vi "Gen - Polar Plot.vi"(4 "Lines/Points":enum16{"Lines", "Points"}(ring)=enum."Points", 5 "font":T1={"desired font(Application) "=enum."Application Font", "[user-specified font] "={"Font Name:"="", "Size"=0, "Strikeout?"=FALSE, "Italic?"=FALSE, "Underline?"=FALSE, "Outline?"=FALSE, "Shadow?"=FALSE, "Bold?"=FALSE}}, 6 "polar attributes":T2={"maximum"=0.0, "minimum"=0.0, "clip to min"=FALSE, "log?(F)"=FALSE, "grid color"=6710886, "plot color"=16711680, "fmt and prec"={"format"=enum."Decimal", "precision"=0}, "visible section"=8} {"minimum" format="%0.3f"; "maximum" format="%0.3f"}, 7 "Size":u16=1, 8 "Scale atrributes":cluster{"Scale Polar plot":dbl, "1 rev FS":dbl}={"Scale Polar plot"=0.2, "1 rev FS"=0.0} {"1 rev FS" format="%#_13g"; "Scale Polar plot" format="%#_13g"}, 9 "dimensions (w,h)":cluster{"width":i16, "height":i16}, 10 "data array [mag, phase (deg)]":cluster{"magnitude":dbl, "phase":dbl}[](array[cluster]) {"phase" format="%0.2f"; "magnitude" format="%0.2f"}, 11 "picture":picture) -> (3 "new picture":picture)   [LabVIEW 2020]
panel:
  in  "top left point(0, 0)":cluster{"x":i16, "y":i16}
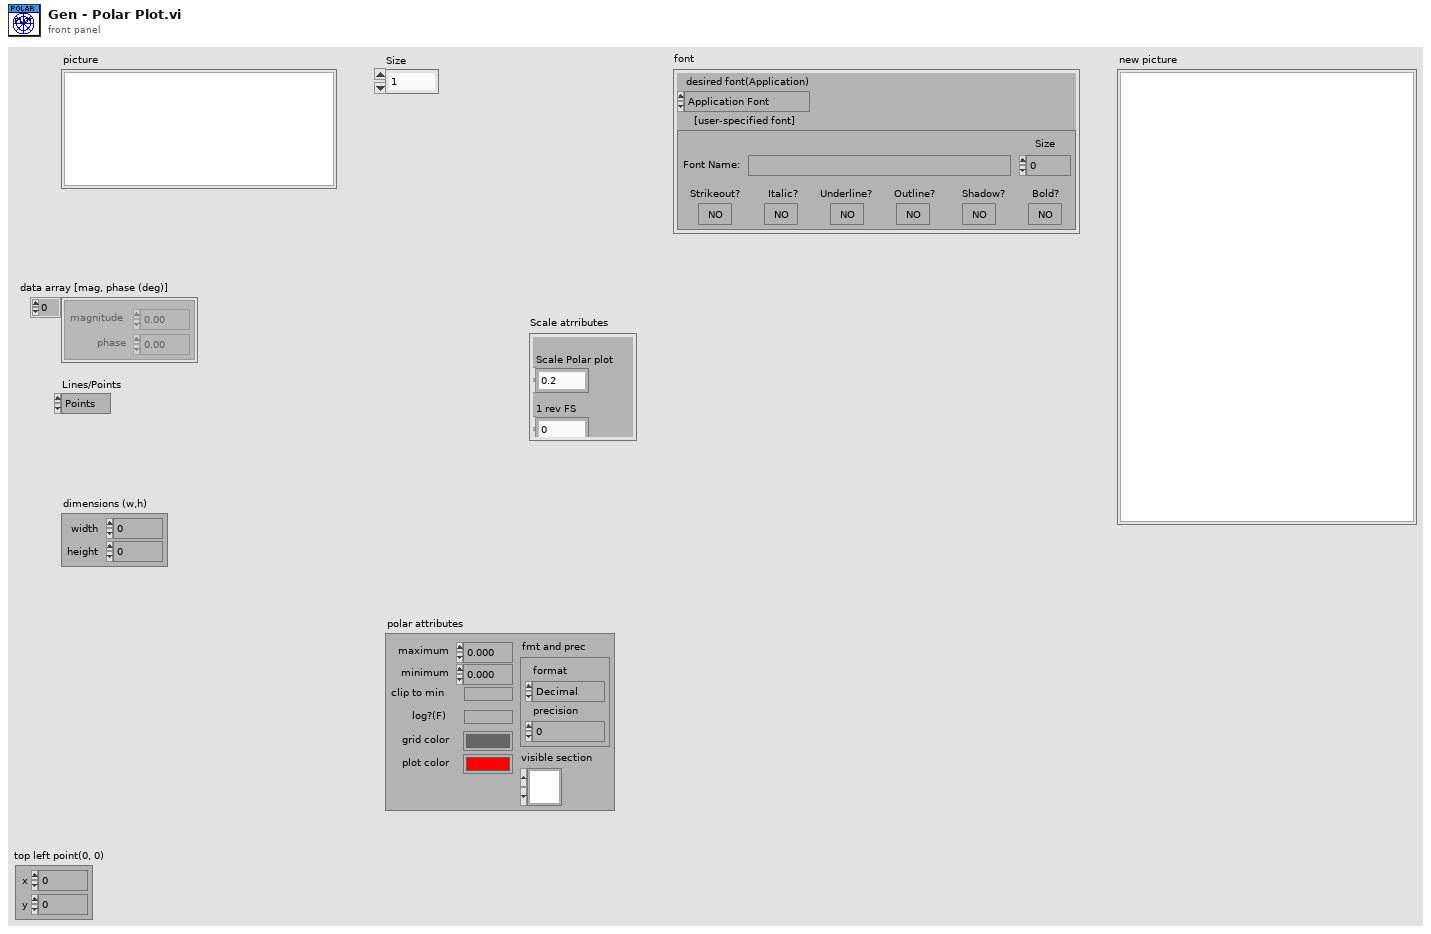
[diagram p1: front panel]
types:
  T1 = cluster{"desired font(Application) ":enum16{"User-specified Font", "Application Font", "System Font", "Dialog Font"}, "[user-specified font] ":cluster{"Font Name:":string, "Size":i16, "Strikeout?":bool, "Italic?":bool, "Underline?":bool, "Outline?":bool, "Shadow?":bool, "Bold?":bool}}
  T2 = cluster{"maximum":dbl, "minimum":dbl, "clip to min":bool, "log?(F)":bool, "grid color":u32, "plot color":u32, "fmt and prec":cluster{"format":enum8{"Decimal", "Scientific", "Engineering", "Binary", "Octal", "Hex"}, "precision":u8}, "visible section":u16}
  T3 = enum16{"User-specified Font", "Application Font", "System Font", "Dialog Font"}
  T4 = cluster{"Font Name:":string, "Size":i16, "Strikeout?":bool, "Italic?":bool, "Underline?":bool, "Outline?":bool, "Shadow?":bool, "Bold?":bool}
  T5 = cluster{"left":i16, "top":i16, "right":i16, "bottom":i16}
  T6 = cluster{"pixel center":cluster{"x":i16, "y":i16}, "scale factors":cluster{"a":dbl, "b":dbl, "log?(F)":bool}, "grid color":u32, "start angle":dbl, "end angle":dbl, "tick length":i16, "pixel radius":i32}
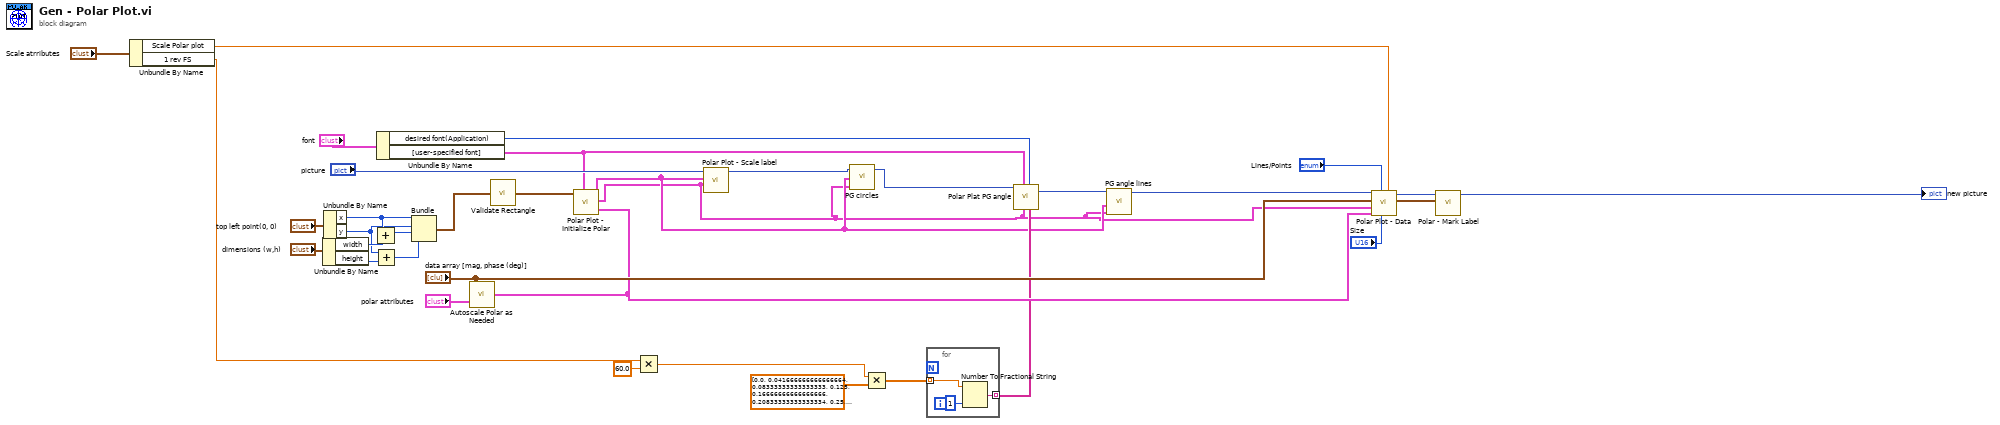
[diagram p0: block diagram]
diagram:
  n1 = Unbundle By Name("Scale atrributes") -> ("Scale Polar plot"=w6:dbl, "1 rev FS"=w5:dbl)
  n2 = Unbundle By Name("dimensions (w,h)") -> ("width"=w34:i16, "height"=w33:i16)
  n3 = Unbundle By Name("top left point(0, 0)") -> ("x"=w32:i16, "y"=w31:i16)
  n4 = Add(x=w32, y=w34) -> (x+y=w30:i16)
  n5 = Add(x=w31, y=w33) -> (x+y=w29:i16)
  n6 = Unbundle By Name("font") -> ("desired font(Application)"=w20:T3, "[user-specified font]"=w3:T4)
  n7 = Bundle("x"=w32, "y"=w31, w30, w29) -> (w28:cluster{"x":i16, "y":i16, i16, i16})  [unwired: 1 in]
  n8 = call <vilib>:"Autoscale Polar as Needed.vi"("polar attributes"="polar attributes", "data"="data array [mag, phase (deg)]") -> ("polar attributes"=w13:T2)
  n9 = call <vilib>:"Validate Rectangle.vi"("rect"=w28) -> ("valid rect"=w14:T5)
  n10 = call "Polar Plot - Initialize Polar.vi"("polar attributes"=w13, "[user-specified font]"=w3, "rect"=w14) -> ("grid measurements"=w1:T6, "scale specs"=w2:cluster{"coordinate":i16, "label":string}[])  [unwired: 7 in]
  n11 = Multiply(x=w5, y=60.0) -> (x*y=w8:dbl)
  n12 = call "Polar Plot - Scale label.vi"("grid measurements"=w1, "scale specs"=w2, "picture"="picture") -> ("new picture"=w15:picture)  [unwired: 8 in]
  n13 = call <vilib>:"PG circles.vi"("picture"=w15, "decade specs"=w2, "grid measurements"=w1) -> ("new picture"=w23:picture)  [unwired: 6 in]
  n14 = Multiply(x=w8, y=dbl[] [0.0, 0.041666666666666664, 0.08333333333333333, 0.125, 0.16666666666666666, 0.20833333333333334, 0.25, 0.2916666666666667, 0.3333333333333333, 0.375, 0.4166666666666667, 0.4583333333333333, 0.5, 0.5416666666666666, 0.5833333333333334, 0.625, 0.6666666666666666, 0.7083333333333334, 0.75, 0.7916666666666666, 0.8333333333333334, 0.875, 0.9166666666666666, 0.9583333333333334, 1.0] ("Array 2")) -> (x*y=w11:dbl[])
  n15 = for {
    tunnel: w11 -> [w39] mode=indexing
    tunnel: [w37] -> w4 mode=indexing
    n16 = Number To Fractional String(number=w39, precision (6)=i16 1) -> (F-format string=w37:string)  [unwired: 2 in]
  }
  n17 = call "Polar Plat PG angle.vi"("axis labels"=w4, "desired font(Application)"=w20, "grid measurements"=w1, "[user-specified font]"=w3, "picture  in"=w23) -> ("picture  out"=w27:picture)  [unwired: 6 in]
  n18 = call <vilib>:"PG angle lines.vi"("grid measurements"=w1, "decade specs"=w2, "picture"=w27) -> ("new picture"=w25:picture)  [unwired: 8 in]
  n19 = call "Polar Plot - Data.vi"("Scale Polar plot"=w6, "Size"="Size", "Lines/Points"="Lines/Points", "polar attributes"=w13, "grid measurements"=w1, "data array [mag, phase (deg)]"="data array [mag, phase (deg)]", "new picture in"=w25) -> ("Position"=w16:cluster{i16, i16}[], "new picture out"=w18:picture)  [unwired: 3 in]
  n20 = call "Polar - Mark Label.vi"("Position"=w16, "new picture in"=w18) -> ("new picture"=→"new picture":picture)  [unwired: 9 in]
